vi "startdelayLUT_checkforchange.vi"() -> (1 "start delay out":variant, 2 "params out":variant[](array[variant]), 3 "go ahead":bool)   [LabVIEW 2012]
doc: "SciScan 1.2 160622"
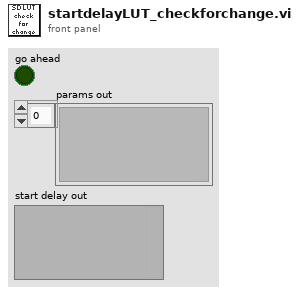
[diagram p1: front panel]
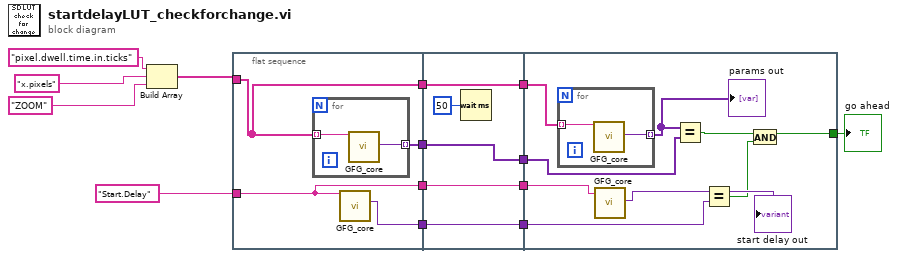
[diagram p0: block diagram]
diagram:
  n1 = Build Array("pixel.dwell.time.in.ticks", "x.pixels", "ZOOM") -> (w11:string[])
  n2 = flat-sequence {
    tunnel: w11 -> [w18]
    tunnel: [w18] -> w9
    tunnel: [w17] -> w7
    tunnel: "Start.Delay" -> [w16]
    tunnel: [w16] -> w3
    tunnel: [w15] -> w2
    tunnel: [w24] -> w10
    tunnel: w9 -> [w24]
    tunnel: [w23] -> w8
    tunnel: w7 -> [w23]
    tunnel: [w22] -> w4
    tunnel: w3 -> [w22]
    tunnel: w2 -> [w21]
    tunnel: [w21] -> w1
    tunnel: [w27] -> w6
    tunnel: w10 -> [w32]
    tunnel: w8 -> [w31]
    tunnel: w4 -> [w30]
    tunnel: w1 -> [w28]
    frame #0 {
      n3 = for {
        tunnel: w18 -> [w20] mode=indexing
        tunnel: [w19] -> w17 mode=indexing
        n4 = call "GFG_core.vi"("Variable Name in"=w20) -> ("Variant Out"=w19:variant)  [unwired: 12 in, 6 out]
      }
      n5 = call "GFG_core.vi"("Variable Name in"=w16) -> ("Variant Out"=w15:variant)  [unwired: 12 in, 6 out]
    }
    frame #1 {
      n6 = Wait (ms)(milliseconds to wait=u32 50) -> ()  [unwired: 1 out]
    }
    frame #2 {
      n7 = for {
        tunnel: [w36] -> w33 mode=indexing
        tunnel: w32 -> [w35] mode=indexing
        n8 = call "GFG_core.vi"("Variable Name in"=w35) -> ("Variant Out"=w36:variant)  [unwired: 12 in, 6 out]
      }
      "params out" <- w33
      n9 = call "GFG_core.vi"("Variable Name in"=w30) -> ("Variant Out"=w29:variant)  [unwired: 12 in, 6 out]
      "start delay out" <- w29
      n10 = Equal?(x=w33, y=w31) -> (x = y?=w34:bool)
      n11 = Equal?(x=w29, y=w28) -> (x = y?=w26:bool)
      n12 = And(x=w34, y=w26) -> (x .and. y?=w27:bool)
    }
  }
  "go ahead" <- w6
